vi "ElevatorSim_CalcK14.vi"(8 "dT_Seconds":dbl=1.0, 9 "U":T3, 10 "current_xHat":T3, 11 "LINEAR_SYSTEM_SIM":T1) -> (3 "updated_xHat":T3)   [LabVIEW 2019, in "Trajectory_Library.lvlib"]
doc: "Creates a new LINEAR SYSTEM data cluster with the specified values. \n\n\nInputs: \n - XXX -- XXX.\n\nOutputs:\n - XXX -- XXX."
uses:
  <vilib>/Analysis/Matrix/Datatypes/RealMatrix.ctl
  LINEAR_SYSTEM_SIM.ctl
  LINEAR_SYSTEM.ctl
  Trajectory_Library.lvlib
  <vilib>/Analysis/Matrix/NI_Matrix.lvlib
panel:
  # "<States, 1>"
  # "<Outputs, 1>"
  # "<Inputs, 1>"
  # "<Outputs, 1>"
  # "<States,States>"
  # "<States,Inputs>"
  # "<Outputs,States>"
  # "<Outputs,Inputs>"
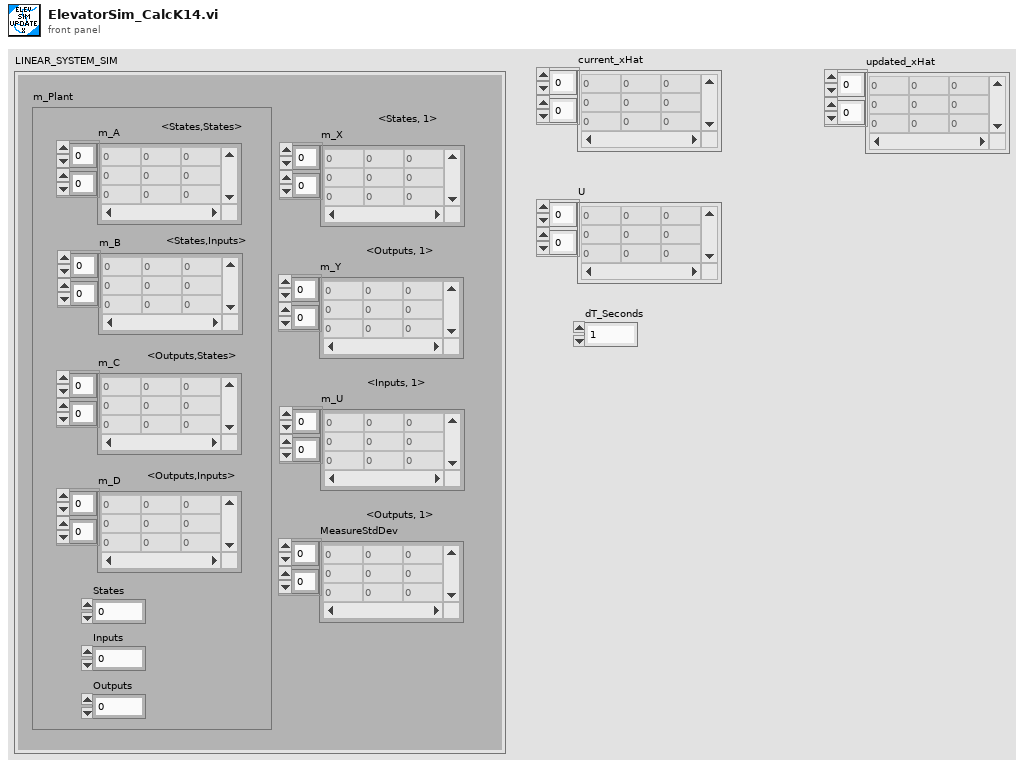
[diagram p1: front panel]
types:
  T1 = typedef "Trajectory_Library.lvlib/LINEAR_SYSTEM_SIM.ctl" = cluster{"m_Plant":T2, "m_X":T3, "m_Y":T3, "m_U":T3, "MeasureStdDev":T3}
  T2 = typedef "Trajectory_Library.lvlib/LINEAR_SYSTEM.ctl" = cluster{"m_A":T3, "m_B":T3, "m_C":T3, "m_D":T3, "States":i32, "Inputs":i32, "Outputs":i32}
  T3 = typedef "NI_Matrix.lvlib/RealMatrix.ctl" = dbl[][]
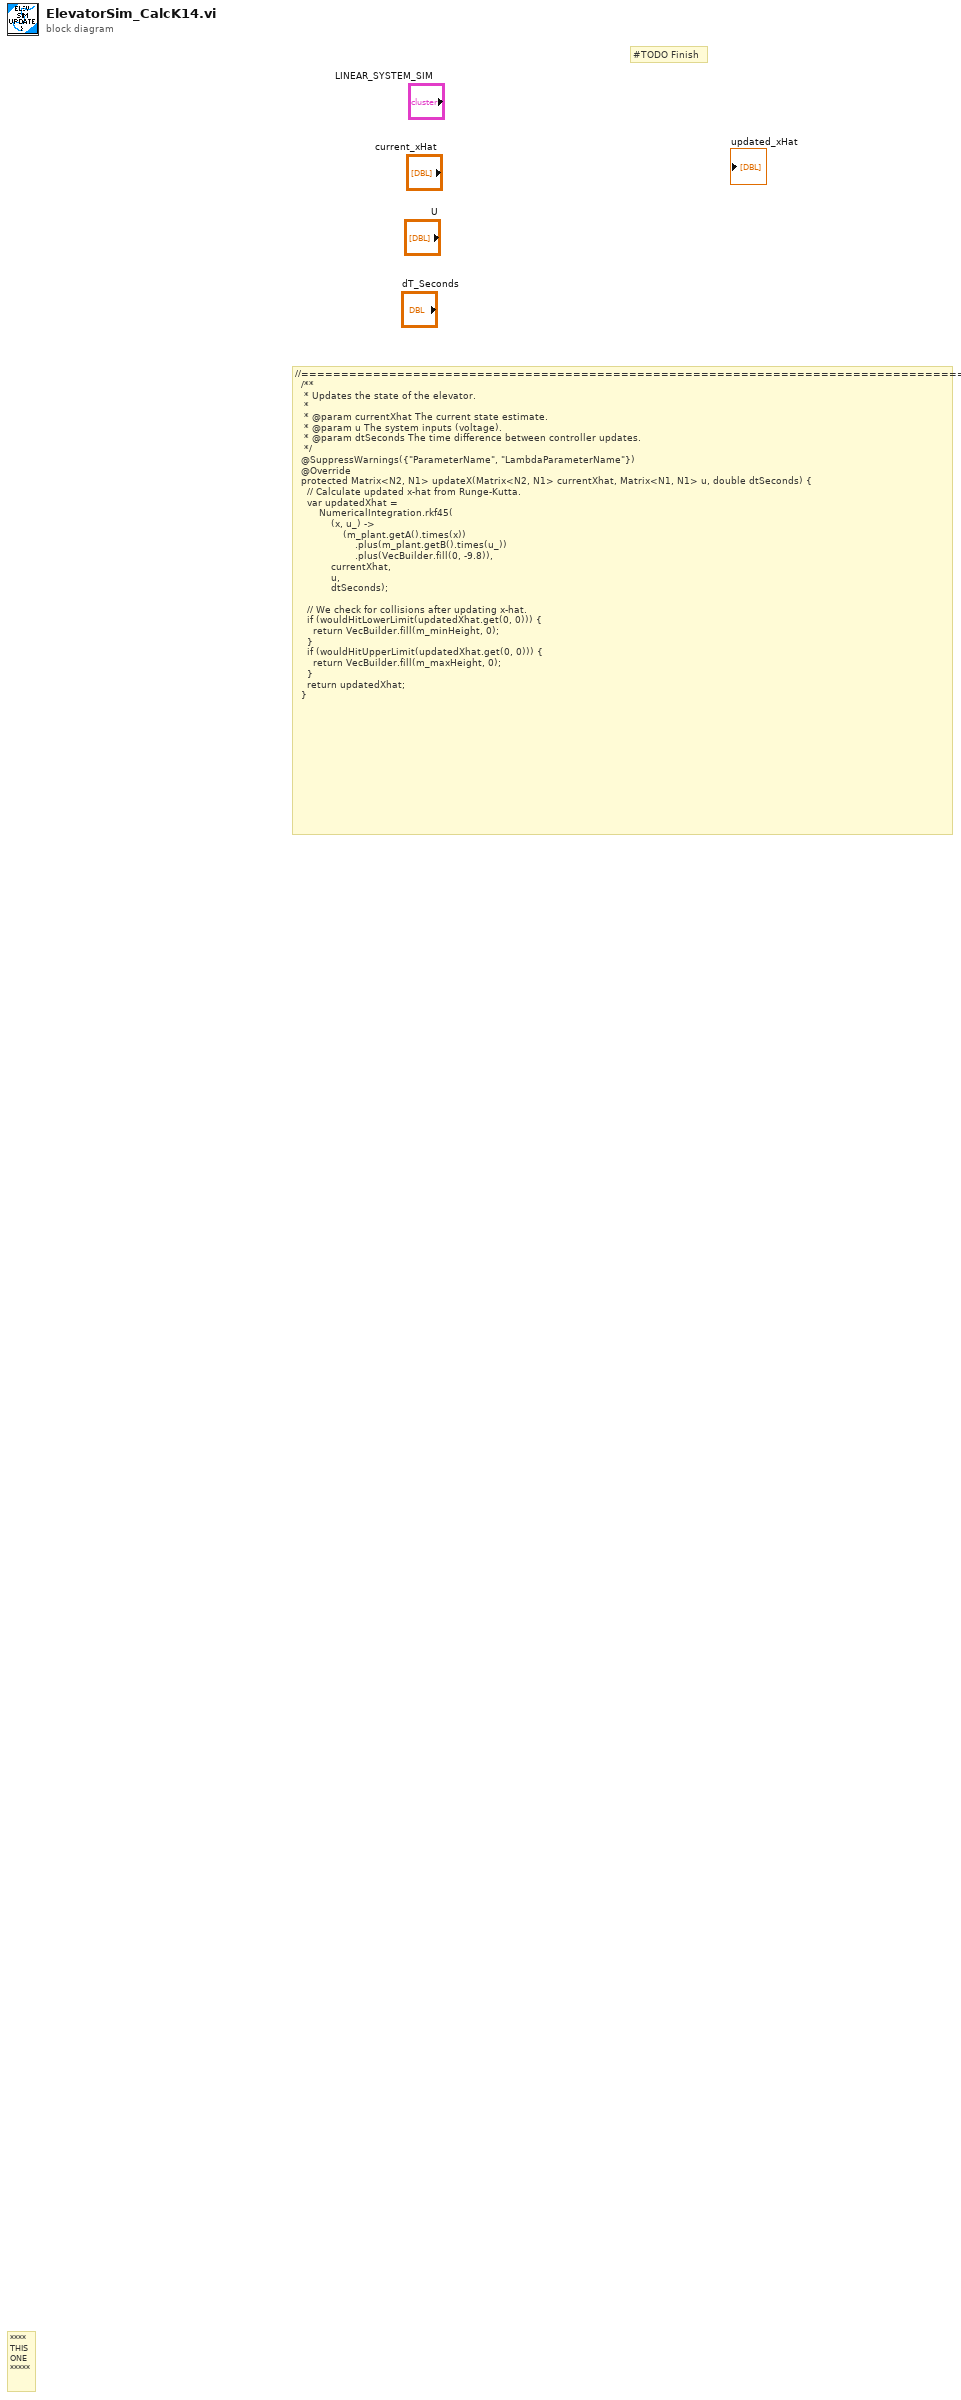
[diagram p0: block diagram]
diagram:
  # "#TODO Finish"
  # "//===================================================================================\n  /**\n   * Updates the state of the elevator.\n   *\n   * @param currentXhat The current state estimate.\n   * @param u The system inputs (voltage).\n   * @param dtSeconds The time difference between controller updates.\n   */\n  @SuppressWarnings({\"ParameterName\", \"LambdaParameterName\"})\n  @Override\n  protected Matrix<N2, N1> updateX(Matrix<N2, N1> currentXhat, Matrix<N1, N1> u, double dtSeconds) {\n    // Calculate updated x-hat from Runge-Kutta.\n    var updatedXhat =\n        NumericalIntegration.rkf45(\n            (x, u_) ->\n                (m_plant.getA().times(x))\n                    .plus(m_plant.getB().times(u_))\n                    .plus(VecBuilder.fill(0, -9.8)),\n            currentXhat,\n            u,\n            dtSeconds);\n\n    // We check for collisions after updating x-hat.\n    if (wouldHitLowerLimit(updatedXhat.get(0, 0))) {\n      return VecBuilder.fill(m_minHeight, 0);\n    }\n    if (wouldHitUpperLimit(updatedXhat.get(0, 0))) {\n      return VecBuilder.fill(m_maxHeight, 0);\n    }\n    return updatedXhat;\n  }"
  # "****\nTHIS\nONE\n*****"
